vi "chart series set error bars.vi"(8 "error in (no error)":errorcluster, 9 "value":dbl, 10 "type":u8, 11 "error_bars":u32) -> (0 "error out":errorcluster)   [LabVIEW 8.6]
doc: "void chart_series_set_error_bars(lxw_series_error_bars error_bars, uint8_t type, double value);"
uses:
  pending_lvxlsxwriter/xlsxwriter.dll
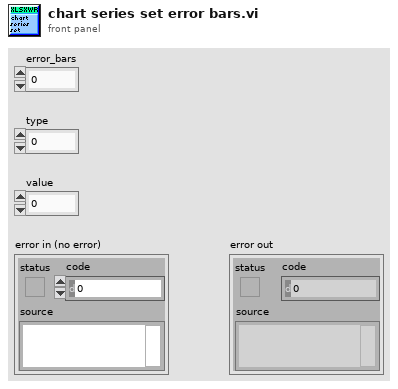
[diagram p1: front panel]
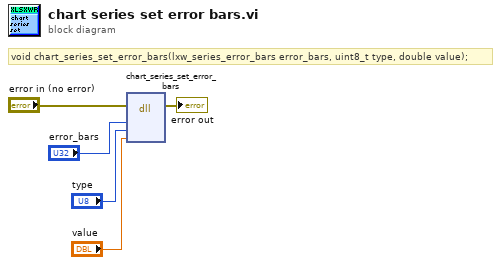
[diagram p0: block diagram]
diagram:
  # "void chart_series_set_error_bars(lxw_series_error_bars error_bars, uint8_t type, double value);"
  n1 = dll-call lib="C:/Users/WDAGUtilityAccount/Desktop/pending_lvxlsxwriter/xlsxwriter.*" fn="chart_series_set_error_bars"(error in="error in (no error)", "error_bars"="error_bars", "type"="type", "value"="value") -> (error out=→"error out":errorcluster)  [unwired: 6 in, 1 out]
